vi "Logging_2.vi"(8 "error in":errorcluster, 9 "Filename":path=path "C:/1. Rocket Research Project/CollectedData/Plots/TestingData.lvm", 10 "Enable":bool=TRUE, 11 "output cluster":T1) -> (0 "error out":errorcluster)   [LabVIEW 2022 SP3]
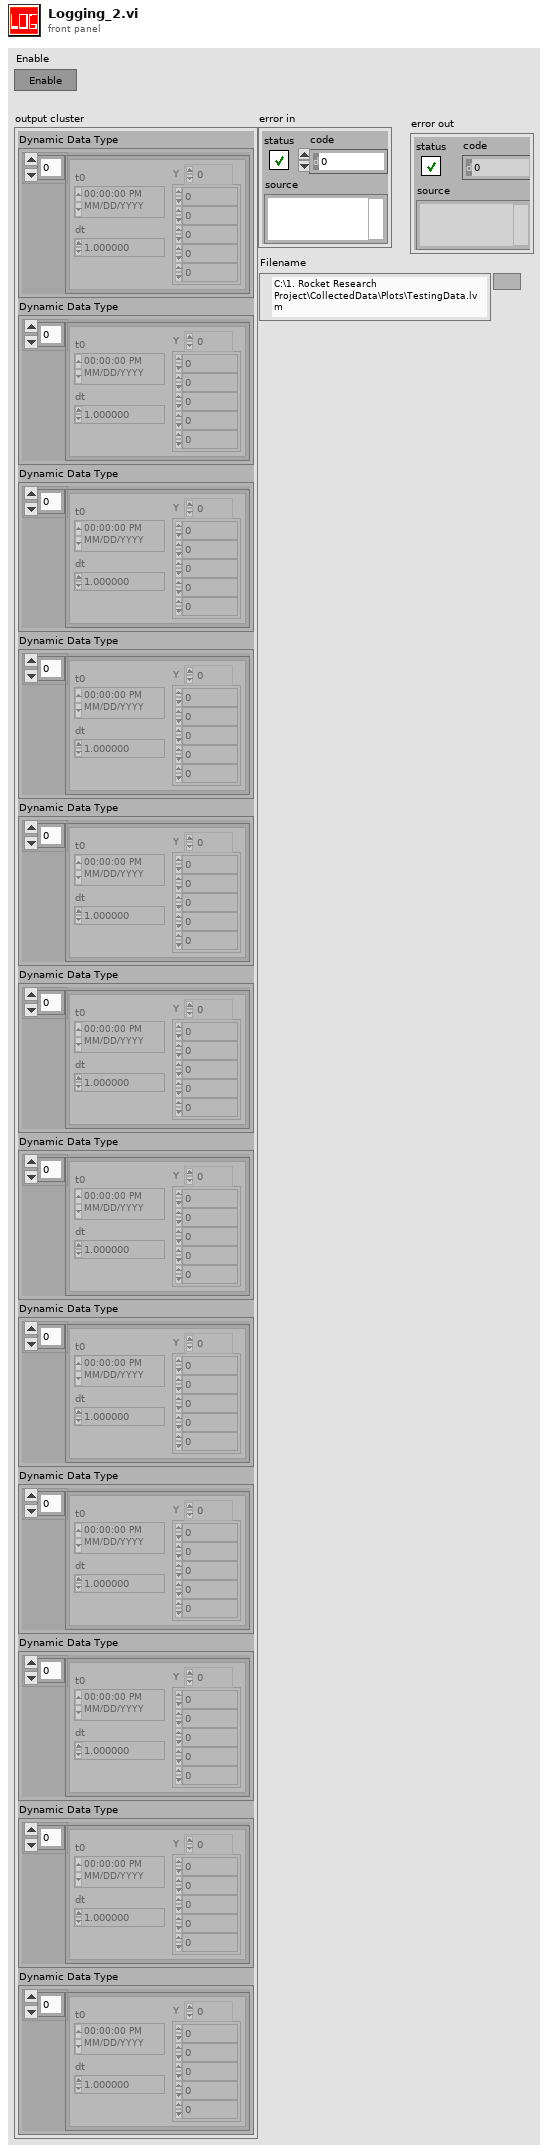
[diagram p1: front panel]
types:
  T1 = cluster{"Dynamic Data Type":dynamicdata, "Dynamic Data Type":dynamicdata, "Dynamic Data Type":dynamicdata, "Dynamic Data Type":dynamicdata, "Dynamic Data Type":dynamicdata, "Dynamic Data Type":dynamicdata, "Dynamic Data Type":dynamicdata, "Dynamic Data Type":dynamicdata, "Dynamic Data Type":dynamicdata, "Dynamic Data Type":dynamicdata, "Dynamic Data Type":dynamicdata, "Dynamic Data Type":dynamicdata}
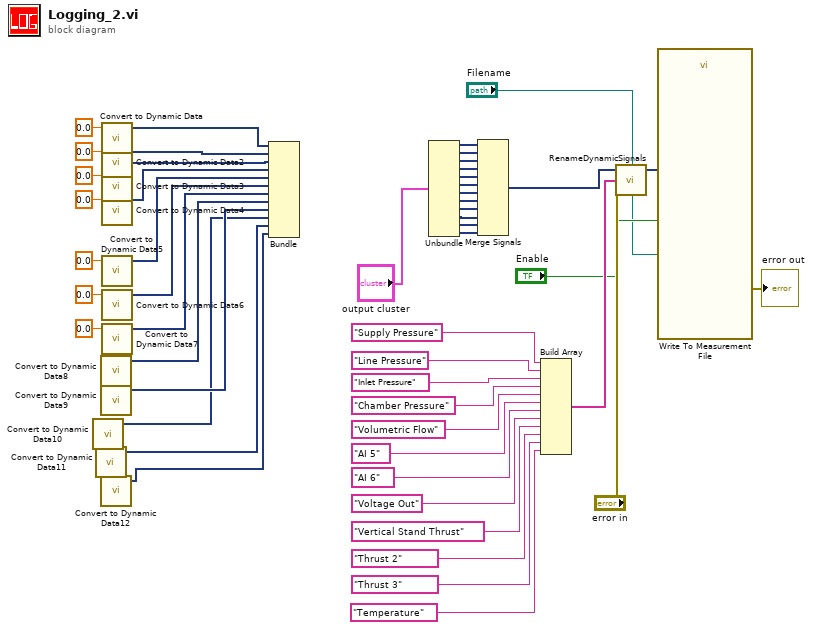
[diagram p0: block diagram]
diagram:
  n1 = call "Convert to Dynamic Data10"() -> ("Dynamic Data Type"=w34:dynamicdata)  [unwired: 4 in]
  n2 = call "Convert to Dynamic Data11"() -> ("Dynamic Data Type"=w33:dynamicdata)  [unwired: 4 in]
  n3 = call "Convert to Dynamic Data8"() -> ("Dynamic Data Type"=w36:dynamicdata)  [unwired: 4 in]
  n4 = call "Convert to Dynamic Data9"() -> ("Dynamic Data Type"=w35:dynamicdata)  [unwired: 4 in]
  n5 = call "Convert to Dynamic Data12"() -> ("Dynamic Data Type"=w32:dynamicdata)  [unwired: 4 in]
  n6 = call "Convert to Dynamic Data"("Double"=0.0) -> ("Dynamic Data Type"=w48:dynamicdata)  [unwired: 3 in]
  n7 = call "Convert to Dynamic Data2"("Double"=0.0) -> ("Dynamic Data Type"=w47:dynamicdata)  [unwired: 3 in]
  n8 = call "Convert to Dynamic Data3"("Double"=0.0) -> ("Dynamic Data Type"=w41:dynamicdata)  [unwired: 3 in]
  n9 = call "Convert to Dynamic Data4"("Double"=0.0) -> ("Dynamic Data Type"=w40:dynamicdata)  [unwired: 3 in]
  n10 = call "Convert to Dynamic Data5"("Double"=0.0) -> ("Dynamic Data Type"=w39:dynamicdata)  [unwired: 3 in]
  n11 = call "Convert to Dynamic Data6"("Double"=0.0) -> ("Dynamic Data Type"=w38:dynamicdata)  [unwired: 3 in]
  n12 = call "Convert to Dynamic Data7"("Double"=0.0) -> ("Dynamic Data Type"=w37:dynamicdata)  [unwired: 3 in]
  n13 = Bundle("Dynamic Data Type"=w48, "Dynamic Data Type"=w47, "Dynamic Data Type"=w41, "Dynamic Data Type"=w40, "Dynamic Data Type"=w39, "Dynamic Data Type"=w38, "Dynamic Data Type"=w37, "Dynamic Data Type"=w36, "Dynamic Data Type"=w35, "Dynamic Data Type"=w34, "Dynamic Data Type"=w33, "Dynamic Data Type"=w32) -> ()  [unwired: 1 in, 1 out]
  n14 = Unbundle("output cluster") -> ("Dynamic Data Type"=w19:dynamicdata, "Dynamic Data Type"=w20:dynamicdata, "Dynamic Data Type"=w21:dynamicdata, "Dynamic Data Type"=w22:dynamicdata, "Dynamic Data Type"=w23:dynamicdata, "Dynamic Data Type"=w24:dynamicdata, "Dynamic Data Type"=w25:dynamicdata, "Dynamic Data Type"=w26:dynamicdata, "Dynamic Data Type"=w27:dynamicdata, "Dynamic Data Type"=w28:dynamicdata, "Dynamic Data Type"=w29:dynamicdata, "Dynamic Data Type"=w30:dynamicdata)
  n15 = Merge Signals(w19, w20, w21, w22, w23, w24, w25, w26, w27, w28, w29, w30) -> (w18:dynamicdata)
  n16 = Build Array("Supply Pressure", "Line Pressure", "Inlet Pressure", "Chamber Pressure", "Volumetric Flow", "AI 5", "AI 6", "Voltage Out" ("element"), "Vertical Stand Thrust", "Thrust 2", "Thrust 3", "Temperature") -> (w5:string[])
  n17 = call "RenameDynamicSignals.vi"("error in"="error in", "New Signal Names"=w5, "Dynamic Data In"=w18) -> ("Dynamic Data Out"=w51:dynamicdata)  [unwired: 1 in, 1 out]
  n18 = call "Write To Measurement File"("Signals"=w51, "Enable"="Enable", "Filename"="Filename") -> ("error out"=→"error out":errorcluster)  [unwired: 14 in, 2 out]
